vi "Actor Core.vi"(8 "error in":errorcluster, 11 "Gage digitizer actor in":refnum<class "Gage digitizer actor.lvclass">) -> (0 "error out":errorcluster, 3 "Actor out":refnum<class "Actor.lvclass">)   [LabVIEW 2015, in "Gage digitizer actor.lvclass"]
doc: "(<B>Filename</B>: Actor Framework.lvlib:Actor.lvclass:Actor Core.vi)\n\nReceives messages to the actor, reacts to them, and initiates any error handling that may shut the actor down.\n\nDescendant classes may override this VI to append parallel tasks for the actor to complete while it handles messages. Overrides use the Call Parent Method node."
uses:
  Gage digitizer actor.lvclass
  <vilib>/ActorFramework/Actor/Actor.lvclass
  Basic controlls.ctl
  Gage digitizer actor.lvclass/Gage digitizer actor.ctl
  <vilib>/ActorFramework/Actor/Actor.lvclass/Actor.ctl
  <vilib>/ActorFramework/Message Enqueuer/Message Enqueuer.lvclass/Message Enqueuer.ctl
  <vilib>/Analysis/baseanly.llb/Mean (DBL).vi
  <vilib>/ActorFramework/Message Enqueuer/Init from Existing Queue.vi
  <vilib>/ActorFramework/Message Enqueuer/Enqueue.vi
  <vilib>/ActorFramework/Message Priority Queue/Priority Enqueue.vi
  <vilib>/ActorFramework/Message Enqueuer/Message Enqueuer.lvclass
  <vilib>/ActorFramework/Stop Msg/Stop Msg.lvclass
  Initialize request message/Initialize request msg.lvclass
  Acquire data request message/Acquire data msg.lvclass
  <vilib>/Analysis/NI_AALBase.lvlib
panel:
  in  "Average data":i16[][](array[numeric])
  in  "Numer to average":i16=5
  in  "Average data?":bool
  in  "Path":path=path "C:/GitHub/PulseEcho/Data/TestData/data.bin"
  in  "Save data?":bool=TRUE
  in  "Numeric Control":i32=-1
  in  "Refresh Button":bool
  out "Waveform Graph":waveform(dbl)(graph)
  in  "Acquire data":bool
  in  "Control cluster":T1={"Number of points"=101600.0, "Input Range"=200, "Trigger Level"=26, "Trigger source"=TRUE} {"Trigger Level" min=-100 max=100 step=1 scale=-60.0..60.0; "Input Range" items=["+/- 5 V"=10000, "+/- 2 V"=4000, "+/- 1 V"=2000, "+/- 500 mV"=1000, "+/- 200 mV"=400, "+/- 100 mV"=200]; "Number of points" min=160.0 step=160.0}
  in  "Stop Button":bool
  # "Program Controls"
  # "Basic Card Controls"
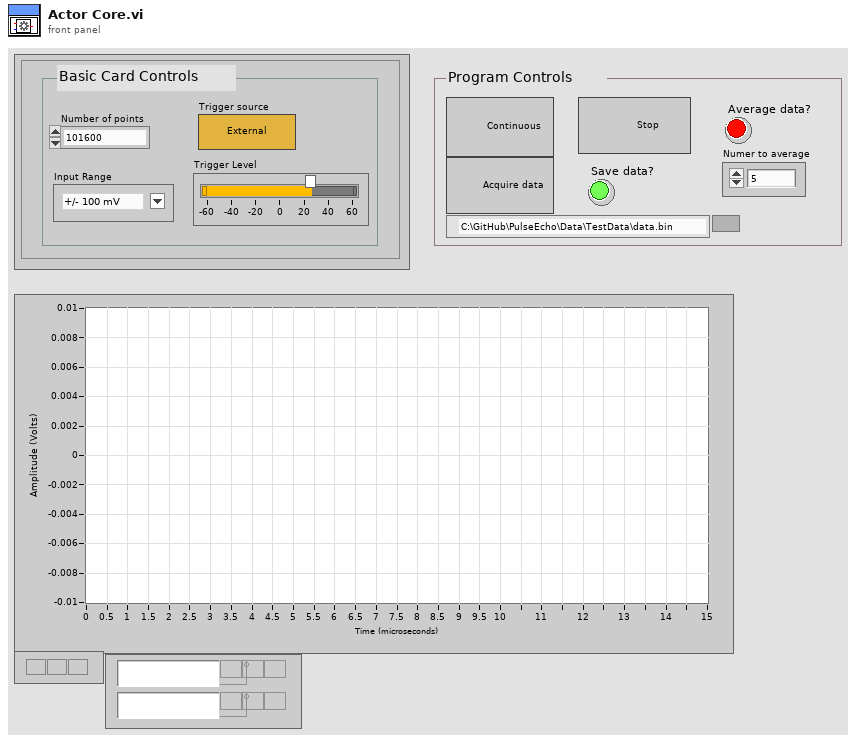
[diagram p1: front panel]
types:
  T1 = typedef "Basic controlls.ctl" = cluster{"Number of points":dbl, "Input Range":u32, "Trigger Level":i32, "Trigger source":bool}
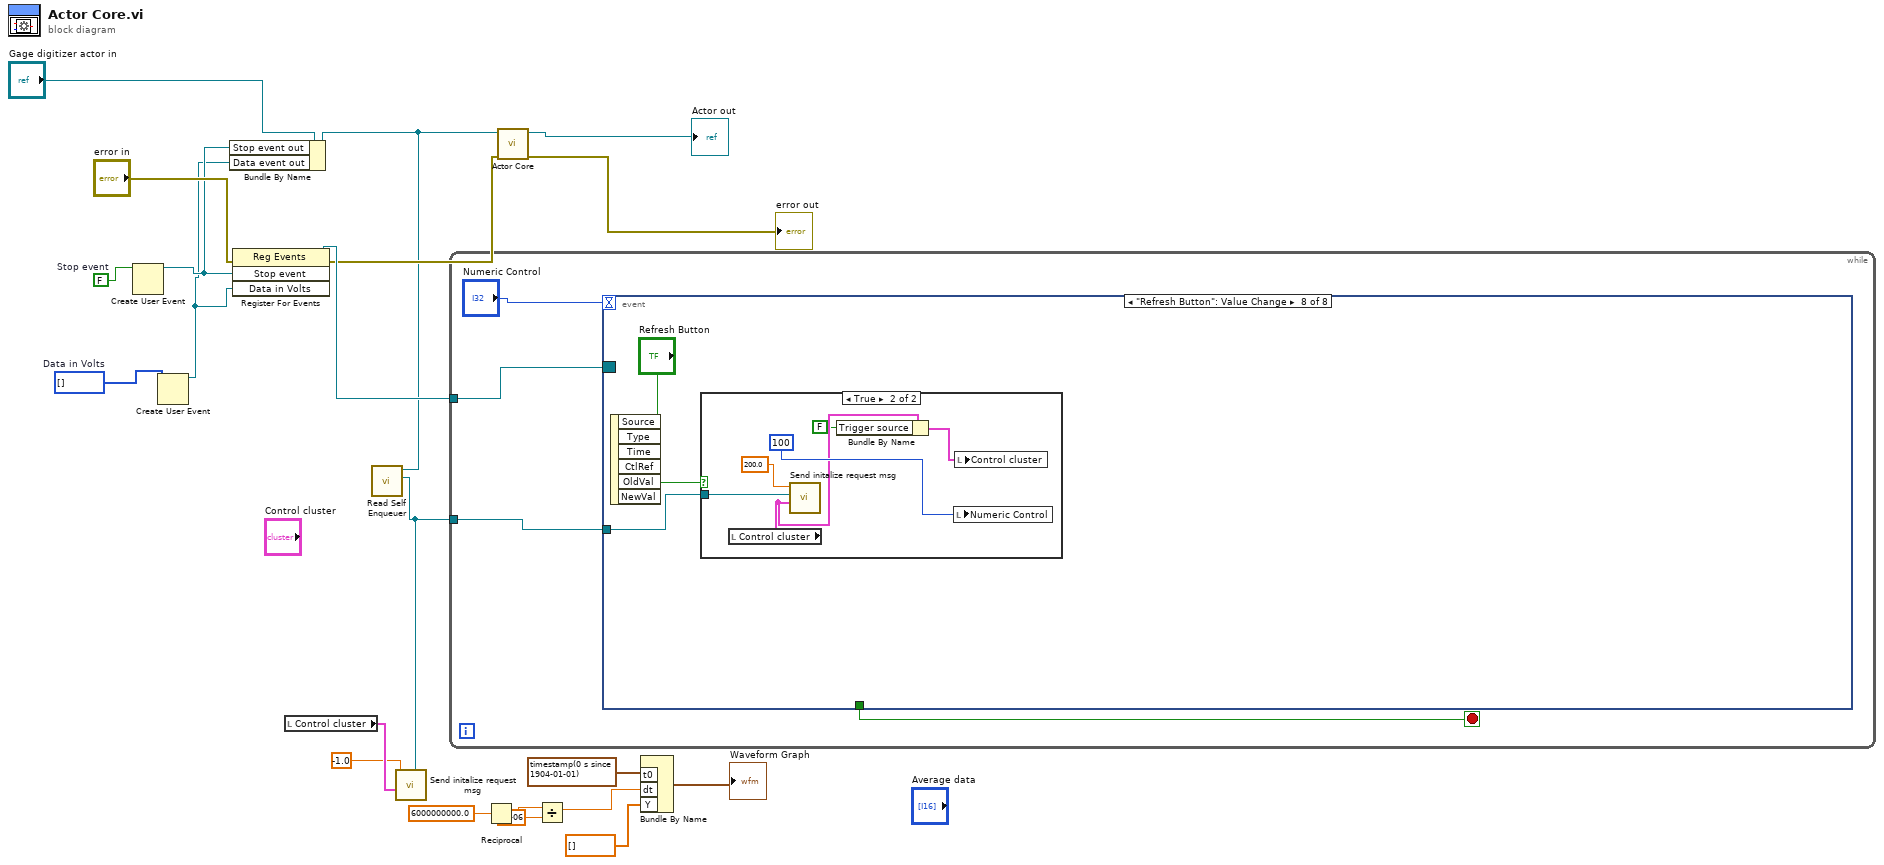
[diagram p0: block diagram]
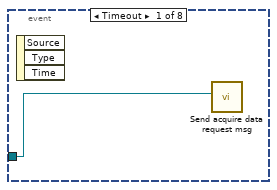
[diagram p2: hidden frame]
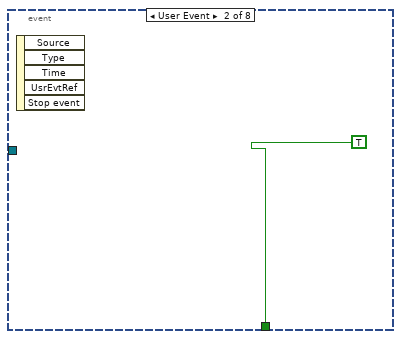
[diagram p3: hidden frame]
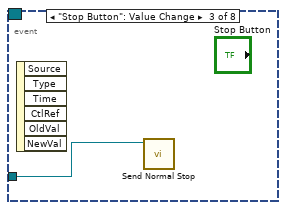
[diagram p4: hidden frame]
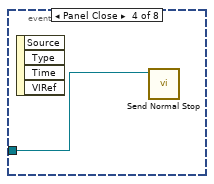
[diagram p5: hidden frame]
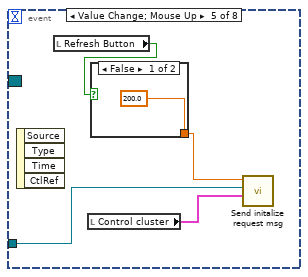
[diagram p6: hidden frame]
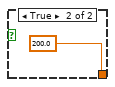
[diagram p7: hidden frame]
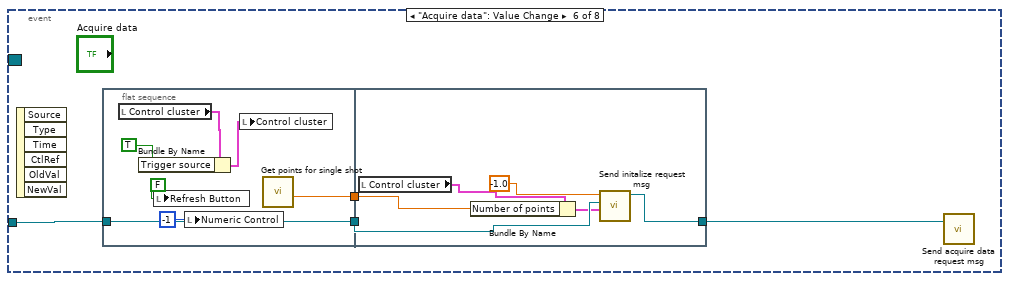
[diagram p8: hidden frame]
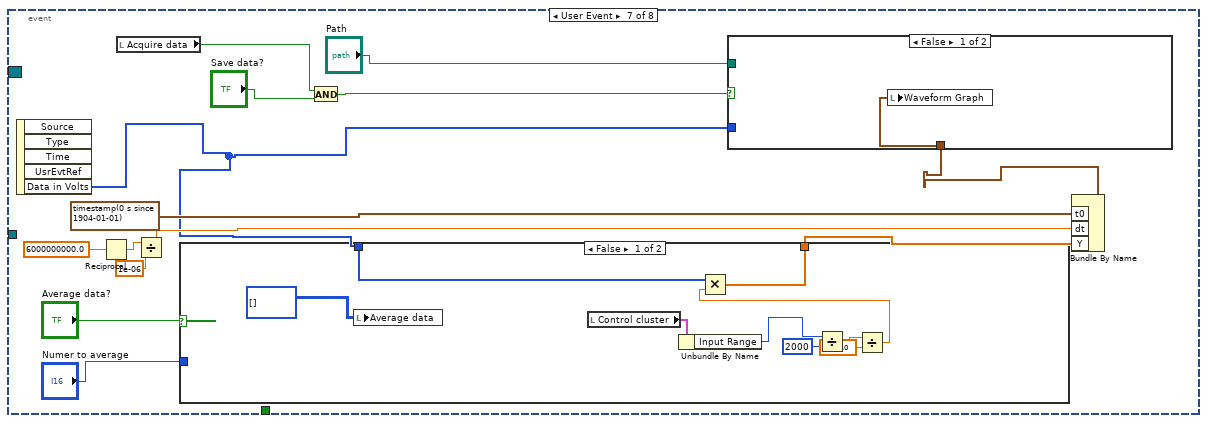
[diagram p9: hidden frame]
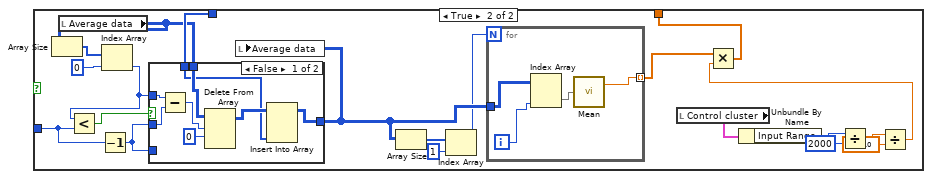
[diagram p10: hidden frame]
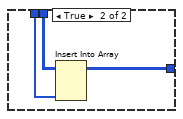
[diagram p11: hidden frame]
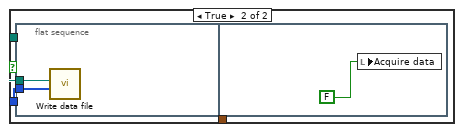
[diagram p12: hidden frame]
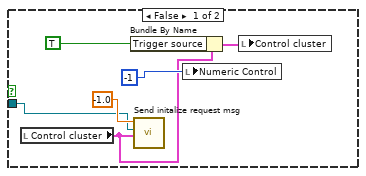
[diagram p13: hidden frame]
diagram:
  w12 = i16[] []  # Data in Volts
  w19 = FALSE  # Stop event
  n1 = Create User Event(user event datatype=w19) -> (user event=w16:refnum<user-event>)  [unwired: 1 in, 1 out]
  n2 = Create User Event(user event datatype=w12) -> (user event=w2:refnum<user-event>)  [unwired: 1 in, 1 out]
  n3 = Bundle By Name(cluster="Gage digitizer actor in", "Stop event out"=w16, "Data event out"=w2) -> (w10:refnum<class "Gage digitizer actor.lvclass">)
  n4 = register-events(error in="error in", w16, w2) -> (reference out=w18:refnum<event-registration>, error out=w17:errorcluster)  [unwired: 1 in]
  n5 = local read "Control cluster"() -> (w13:T1)
  n6 = call <vilib>:"Read Self Enqueuer.vi"("Actor"=w10) -> ("Self Enqueuer"=w14:refnum<class "Message Enqueuer.lvclass">)  [unwired: 10 in]
  n7 = call "Send initalize request msg.vi"("Trigger Timeout (10000000)"=-1.0, "Message Enqueuer in"=w14, "Control cluster"=w13) -> ()  [unwired: 6 in, 2 out]
  n8 = while {
    tunnel: w18 -> [w25]
    tunnel: w14 -> [w23]
    stop <- w24 stop-if-true
    n9 = event shown="[7] \"Refresh Button\": Value Change" {
      selector: w25 -> [_ _ _ _ _ _ _ _]
      dyn-events: _ -> [_ _ _ _ _ _ _ _]
      timeout: "Numeric Control" -> [_ _ _ _ _ _ _ _]
      tunnel: [_ TRUE _ _ _ _ _ _] -> w24
      tunnel: w23 -> [w26 _ w28 w29 w33 w39 _ w118]
      event Timeout {
        n10 = event-data() -> ()  [unwired: 1 in, 3 out]
        n11 = call "Send acquire data request msg.vi"("Message Enqueuer in"=w26) -> ()  [unwired: 8 in, 2 out]
      }
      event User Event {
        n12 = event-data() -> ()  [unwired: 1 in, 5 out]
      }
      event "Stop Button": Value Change {
        n13 = event-data() -> ()  [unwired: 1 in, 6 out]
        n14 = call <vilib>:"Send Normal Stop.vi"("Message Enqueuer"=w28) -> ()  [unwired: 10 in, 1 out]
      }
      event Panel Close {
        n15 = event-data() -> ()  [unwired: 1 in, 4 out]
        n16 = call <vilib>:"Send Normal Stop.vi"("Message Enqueuer"=w29) -> ()  [unwired: 10 in, 1 out]
      }
      event Value Change; Mouse Up {
        n17 = event-data() -> ()  [unwired: 1 in, 4 out]
        n18 = local read "Refresh Button"() -> (w30:bool)
        n19 = local read "Control cluster"() -> (w32:T1)
        n20 = case shown="False" w30 {
          tunnel: [200.0 ("Trigger Timeout (10000000)") 200.0 ("Trigger Timeout (10000000)")] -> w31
          frame False {
          }
          frame True {
          }
        }
        n21 = call "Send initalize request msg.vi"("Trigger Timeout (10000000)"=w31, "Message Enqueuer in"=w33, "Control cluster"=w32) -> ()  [unwired: 6 in, 2 out]
      }
      event "Acquire data": Value Change {
        n22 = event-data() -> ()  [unwired: 1 in, 6 out]
        n23 = flat-sequence {
          tunnel: w39 -> [w46]
          tunnel: [w46] -> w38
          tunnel: [w44] -> w37
          tunnel: w38 -> [w51]
          tunnel: w37 -> [w48]
          tunnel: [w52] -> w36
          frame #0 {
            n24 = local read "Control cluster"() -> (w42:T1)
            n25 = Bundle By Name(cluster=w42, "Trigger source"=TRUE) -> (w40:T1)
            n26 = local write "Refresh Button"(FALSE ("Refresh Button")) -> ()
            n27 = local write "Numeric Control"(-1 ("Numeric Control")) -> ()
            n28 = local write "Control cluster"(w40) -> ()
            n29 = call "Get points for single shot.vi"() -> ("Number of Points 2"=w44:dbl)  [unwired: 9 in, 1 out]
          }
          frame #1 {
            n30 = local read "Control cluster"() -> (w47:T1)
            n31 = Bundle By Name(cluster=w47, "Number of points"=w48) -> (w49:T1)
            n32 = call "Send initalize request msg.vi"("Trigger Timeout (10000000)"=-1.0, "Message Enqueuer in"=w51, "Control cluster"=w49) -> ("Message Enqueuer out"=w52:refnum<class "Message Enqueuer.lvclass">)  [unwired: 6 in, 1 out]
          }
        }
        n33 = call "Send acquire data request msg.vi"("Message Enqueuer in"=w36) -> ()  [unwired: 8 in, 2 out]
      }
      event User Event {
        n34 = event-data() -> ("Data in Volts"=w57:i16[])  [unwired: 1 in, 4 out]
        n35 = Reciprocal(x=6000000000.0) -> (1/x=w64:dbl)
        n36 = local read "Acquire data"() -> (w61:bool)
        n37 = Divide(x=w64, y=1e-06) -> (x/y=w62:dbl)
        n38 = case shown="False" "Average data?" {
          tunnel: w57 -> [w69 w91]
          tunnel: "Numer to average" -> [_ w85]
          tunnel: [w67 w76] -> w54
          frame False {
            n39 = local write "Average data"(i16[][] [] ("Average data 2")) -> ()
            n40 = local read "Control cluster"() -> (w71:T1)
            n41 = Unbundle By Name(w71) -> ("Input Range"=w70:u32)
            n42 = Divide(x=w70, y=u32 2000) -> (x/y=w73:dbl)
            n43 = Divide(x=w73, y=32768.0) -> (x/y=w68:dbl)
            n44 = Multiply(x=w69, y=w68) -> (x*y=w67:dbl[])
          }
          frame True {
            n45 = local read "Average data"() -> (w88:i16[][])
            n46 = Array Size(array=w88) -> (size(s)=w90:i32[])
            n47 = Decrement(x=w85) -> (x-1=w84:i16)
            n48 = Index Array(array=w90, index=0) -> (element=w86:i32)
            n49 = Less?(x=w86, y=w85) -> (x < y?=w87:bool)
            n50 = case shown="False" w87 {
              tunnel: w88 -> [w103 w106]
              tunnel: [w100 w105] -> w95
              tunnel: w91 -> [w101 w104]
              tunnel: w84 -> [_ _]
              tunnel: w86 -> [w99 _]
              tunnel: w84 -> [w98 _]
              frame False {
                n51 = Subtract(x=w99, y=w98) -> (x-y=w96:i32)
                n52 = Delete From Array(array=w103, length=w96, index (row)=0) -> (array with subset deleted=w102:i16[][])  [unwired: 1 in, 1 out]
                n53 = Insert Into Array(array=w102, new element=w101) -> (w100:i16[][])  [unwired: 2 in]
              }
              frame True {
                n54 = Insert Into Array(array=w106, new element=w104) -> (w105:i16[][])  [unwired: 2 in]
              }
            }
            n55 = local write "Average data"(w95) -> ()
            n56 = Array Size(array=w95) -> (size(s)=w94:i32[])
            n57 = Index Array(array=w94, index=1) -> (element=w92:i32)
            n58 = for {
              N: w92 -> [_]
              tunnel: w95 -> [w110]
              tunnel: [w108] -> w78 mode=indexing
              i -> [w107]
              n59 = Index Array(array=w110, index (col)=w107) -> (element=w109:i16[])  [unwired: 1 in]
              n60 = call-poly <vilib>:"Mean.vi"("X"=w109) -> ("mean"=w108:dbl)  [unwired: 1 out]
            }
            n61 = local read "Control cluster"() -> (w83:T1)
            n62 = Unbundle By Name(w83) -> ("Input Range"=w82:u32)
            n63 = Divide(x=w82, y=u32 2000) -> (x/y=w80:dbl)
            n64 = Divide(x=w80, y=32768.0) -> (x/y=w77:dbl)
            n65 = Multiply(x=w78, y=w77) -> (x*y=w76:dbl[])
          }
        }
        n66 = And(x=w61, y="Save data?") -> (x .and. y?=w59:bool)
        n67 = Bundle By Name("t0"=timestamp(0 s since 1904-01-01), "dt"=w62, "Y"=w54) -> (w53:waveform(dbl))  [unwired: 1 in]
        n68 = case shown="False" w59 {
          tunnel: w57 -> [_ w112]
          tunnel: "Path" -> [_ w113]
          tunnel: w53 -> [w111 _]
          frame False {
            n69 = local write "Waveform Graph"(w111) -> ()
          }
          frame True {
            n70 = flat-sequence {
              tunnel: w113 -> [w115]
              tunnel: w112 -> [w114]
              frame #0 {
                n71 = call "Write data file.vi"("Data in Volts"=w114, "Path"=w115) -> ()  [unwired: 9 in, 1 out]
              }
              frame #1 {
                n72 = local write "Acquire data"(FALSE) -> ()
              }
            }
          }
        }
      }
      event "Refresh Button": Value Change {
        n73 = event-data() -> ()  [unwired: 1 in, 6 out]
        n74 = case shown="True" "Refresh Button" {
          tunnel: w118 -> [w123 w130]
          frame False {
            n75 = local read "Control cluster"() -> (w121:T1)
            n76 = Bundle By Name(cluster=w121, "Trigger source"=TRUE) -> (w119:T1)
            n77 = call "Send initalize request msg.vi"("Trigger Timeout (10000000)"=-1.0, "Message Enqueuer in"=w123, "Control cluster"=w121) -> ()  [unwired: 6 in, 2 out]
            n78 = local write "Numeric Control"(-1 ("Timeout")) -> ()
            n79 = local write "Control cluster"(w119) -> ()
          }
          frame True {
            n80 = local read "Control cluster"() -> (w127:T1)
            n81 = call "Send initalize request msg.vi"("Trigger Timeout (10000000)"=200.0, "Message Enqueuer in"=w130, "Control cluster"=w127) -> ()  [unwired: 6 in, 2 out]
            n82 = Bundle By Name(cluster=w127, "Trigger source"=FALSE) -> (w125:T1)
            n83 = local write "Numeric Control"(100 ("Timeout")) -> ()
            n84 = local write "Control cluster"(w125) -> ()
          }
        }
      }
    }
  }
  n85 = Reciprocal(x=6000000000.0) -> (1/x=w7:dbl)
  n86 = call-parent "Actor Core.vi"("error in"=w17, "Actor in"=w10) -> ("error out"=→"error out":errorcluster, "Actor out"=→"Actor out":refnum<class "Actor.lvclass">)  [unwired: 8 in]
  n87 = Divide(x=w7, y=1e-06) -> (x/y=w5:dbl)
  n88 = Bundle By Name("t0"=timestamp(0 s since 1904-01-01), "dt"=w5, "Y"=dbl[] []) -> (→"Waveform Graph":waveform(dbl))  [unwired: 1 in]
